vi "16-ParseNumberOfBITS.vi"(11 "BITS in":bool[](array[boolean])) -> (2 "Number of BITS":u32, 3 "BITS out":bool[](array[boolean]))   [LabVIEW 2019, in "16.lvlib"]
uses:
  16.lvlib
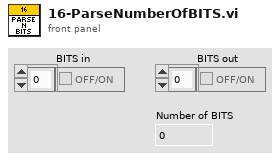
[diagram p1: front panel]
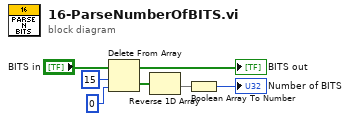
[diagram p0: block diagram]
diagram:
  n1 = Delete From Array(array="BITS in", length=15, index=0) -> (deleted portion=w4:bool[], array with subset deleted=→"BITS out":bool[])
  n2 = Reverse 1D Array(array=w4) -> (reversed array=w3:bool[])
  n3 = Boolean Array To Number(Boolean array=w3) -> (number=→"Number of BITS":u32)
